vi "Find (Create) Object.vi"(7 "Object Path":string, 8 "error in (no error)":errorcluster, 10 "Starting Offset":i32, 11 "JSON":string) -> (0 "error out":errorcluster, 2 "Object offset":i32, 3 "<JSON>":string caption="<JSON> (possibly with empty object inserted)")   [LabVIEW 2015, in "JSONtext.lvlib"]
doc: "Ensures that a JSON Object exists at Path, and returns the offset to that object. If the object does not exist but it's parent object does, then an empty object is inserted. An error is output if a non-object exists at the specified path."
uses:
  JSONtext.lvlib
  Replace at Offset.vi
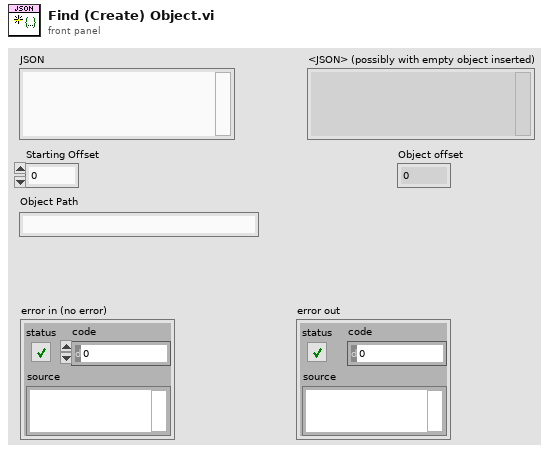
[diagram p1: front panel]
types:
  T1 = typedef "JSONtext.lvlib/Found Items.ctl" = cluster{"Item offset":i32, "Offset past Item":i32, "Name offset":i32, "Offset past Name":i32, "Found":bool, "Empty Object":bool}
  T2 = typedef "JSONtext.lvlib/Parsing State.ctl" = enum16{"Parser Error", "Object", "Array", "String", "Number/Other", "Leading Whitespace", "Object end", "Array end", "Value end"}
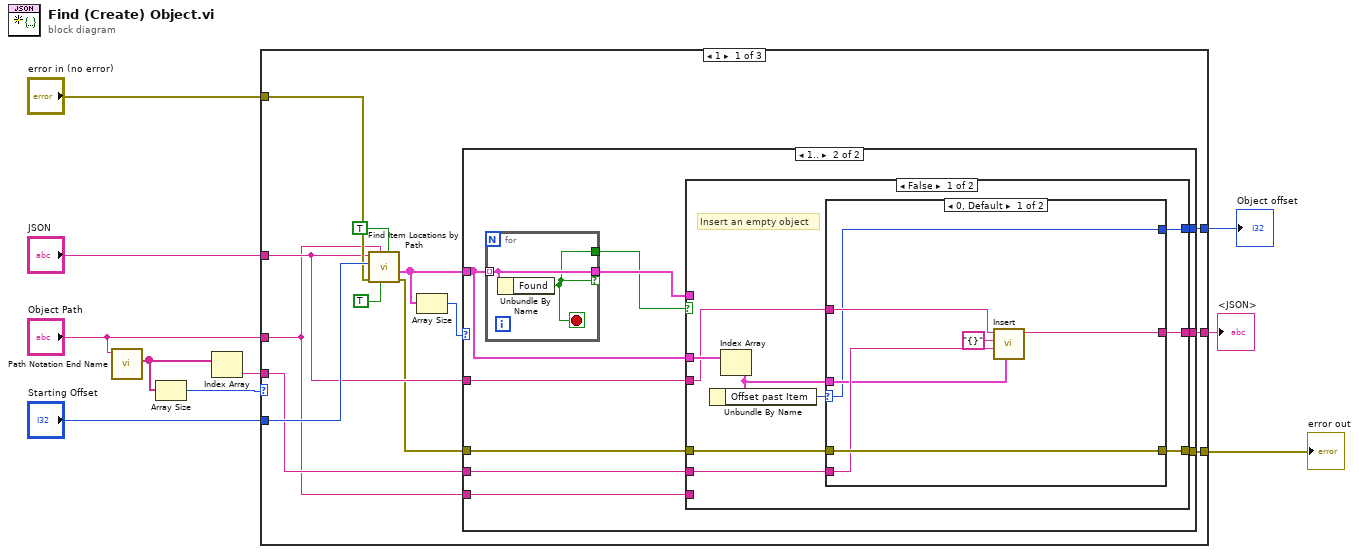
[diagram p0: block diagram]
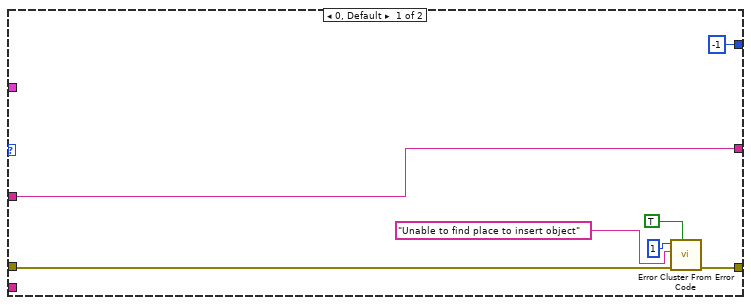
[diagram p2: hidden frame]
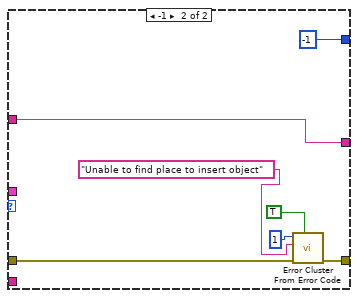
[diagram p3: hidden frame]
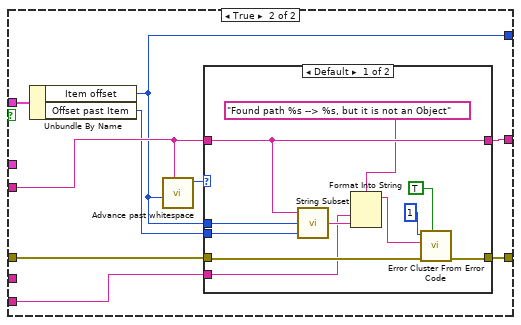
[diagram p4: hidden frame]
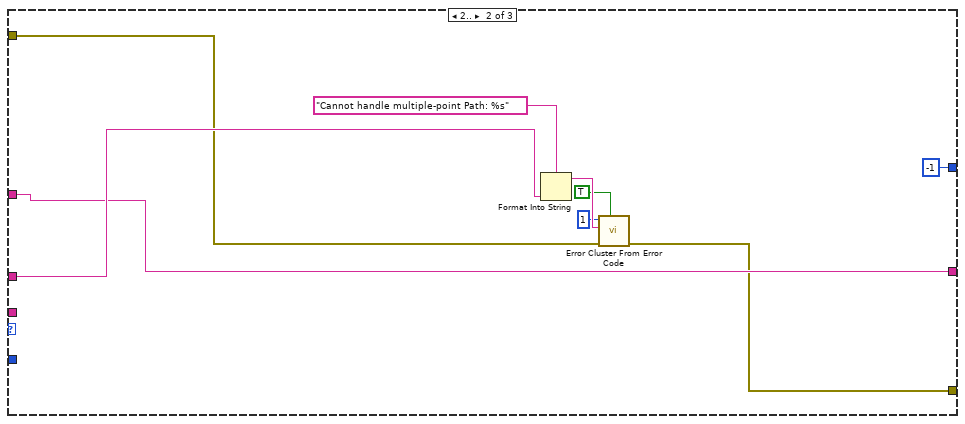
[diagram p6: hidden frame]
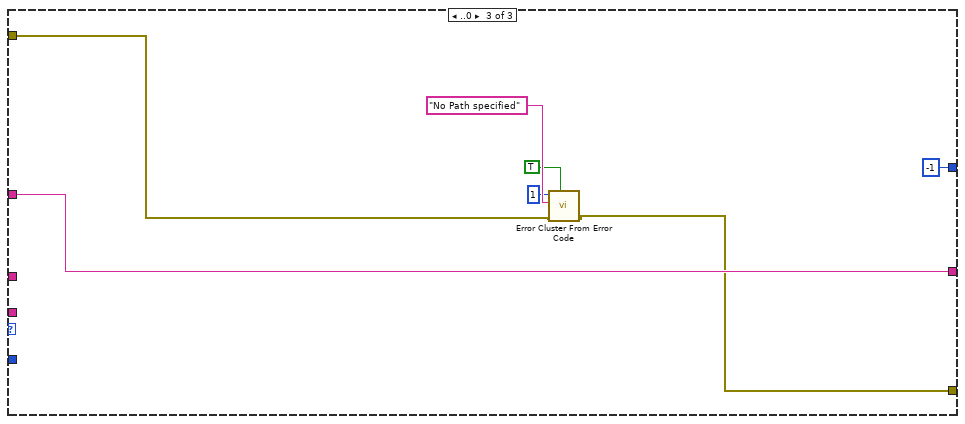
[diagram p7: hidden frame]
diagram:
  n1 = call "Path Notation End Name.vi"("Item Path"="Object Path") -> ("<JSON>End Names"=w5:string[])  [unwired: 10 in]
  n2 = Array Size(array=w5) -> (size(s)=w3:i32)
  n3 = Index Array(array=w5) -> (element=w2:string)  [unwired: 1 in]
  n4 = case shown="1" w3 {
    tunnel: "Object Path" -> [w13 w95 _]
    tunnel: "Starting Offset" -> [w23 _ _]
    tunnel: "error in (no error)" -> [w22 w89 w101]
    tunnel: [w16 w88 w100] -> w8
    tunnel: "JSON" -> [w21 w93 w102]
    tunnel: [w19 -1 ("Item offset") -1 ("Item offset")] -> w6
    tunnel: w2 -> [w15 _ _]
    tunnel: [w14 w93 w102] -> w1
    frame 1 {
      n5 = call "Find Item Locations by Path.vi"("Insertion point if not found"=TRUE, "Only return first found"=TRUE, "Path"=w13, "error in (no error)"=w22, "Object Offset"=w23, "JSON"=w21) -> ("error out"=w17:errorcluster, "Items"=w12:T1[])  [unwired: 4 in]
      n6 = Array Size(array=w12) -> (size(s)=w11:i32)
      n7 = case shown="1.." w11 {
        tunnel: w21 -> [w29 w40]
        tunnel: [-1 ("Item offset") w38] -> w19
        tunnel: w17 -> [w24 w36]
        tunnel: [w25 w35] -> w16
        tunnel: w15 -> [_ w34]
        tunnel: [w29 w33] -> w14
        tunnel: w13 -> [_ w32]
        tunnel: w12 -> [_ w31]
        frame 0, Default {
          n8 = call <vilib>:"Error Cluster From Error Code.vi"("show call chain? (False)"=TRUE, "error in (no error)"=w24, "error message (\"\")"="Unable to find place to insert object", "error code (0)"=1) -> ("error out"=w25:errorcluster)  [unwired: 5 in]
        }
        frame 1.. {
          n9 = for {
            tunnel: w31 -> [w42] mode=indexing
            tunnel: [w42] -> w39 if=w41
            tunnel: [w41] -> w37
            stop <- w41 stop-if-true
            n10 = Unbundle By Name(w42) -> ("Found"=w41:bool)
          }
          n11 = case shown="False" w37 {
            tunnel: w40 -> [w47 w69]
            tunnel: w39 -> [_ w74]
            tunnel: [w43 w68] -> w38
            tunnel: w36 -> [w48 w71]
            tunnel: [w49 w72] -> w35
            tunnel: w31 -> [w51 _]
            tunnel: w34 -> [w46 _]
            tunnel: [w44 w70] -> w33
            tunnel: w32 -> [_ w66]
            frame False {
              # "Insert an empty object"
              n12 = Index Array(array=w51) -> (element=w45:T1)  [unwired: 1 in]
              n13 = Unbundle By Name(w45) -> ("Offset past Item"=w50:i32)
              n14 = case shown="0, Default" w50 {
                selector: w50 -> [w52 _]
                tunnel: [w58 w65] -> w49
                tunnel: w48 -> [w58 w64]
                tunnel: w47 -> [w57 w60]
                tunnel: w46 -> [w56 _]
                tunnel: w45 -> [w54 _]
                tunnel: [w53 w60] -> w44
                tunnel: [w52 -1 ("Item offset")] -> w43
                frame 0, Default {
                  n15 = call "Insert.vi"("Item"=w54, "<JSON>name"=w56, "JSON to Insert"="{}", "JSON in"=w57) -> ("string"=w53:string)  [unwired: 6 in, 1 out]
                }
                frame -1 {
                  n16 = call <vilib>:"Error Cluster From Error Code.vi"("show call chain? (False)"=TRUE, "error in (no error)"=w64, "error message (\"\")"="Unable to find place to insert object", "error code (0)"=1) -> ("error out"=w65:errorcluster)  [unwired: 5 in]
                }
              }
            }
            frame True {
              n17 = Unbundle By Name(w74) -> ("Item offset"=w68:i32, "Offset past Item"=w67:i32)
              n18 = call "Advance past whitespace.vi"("JSON"=w69, "Offset"=w68) -> ("Parser State"=w73:T2)  [unwired: 8 in, 1 out]
              n19 = case shown="Default" w73 {
                tunnel: [w85 w87] -> w72
                tunnel: w71 -> [w84 w87]
                tunnel: [w81 w86] -> w70
                tunnel: w69 -> [w81 w86]
                tunnel: w68 -> [w80 _]
                tunnel: w67 -> [w79 _]
                tunnel: w66 -> [w75 _]
                frame Default {
                  n20 = call "String Subset.vi"("Offset past End"=w79, "Start offset"=w80, "JSON"=w81) -> ("substring"=w77:string)  [unwired: 2 in]
                  n21 = Format Into String(format string="Found path %s --> %s, but it is not an Object" ("error message (\"\")"), w75, w77) -> (resulting string=w76:string)  [unwired: 2 in, 1 out]
                  n22 = call <vilib>:"Error Cluster From Error Code.vi"("show call chain? (False)"=TRUE, "error in (no error)"=w84, "error message (\"\")"=w76, "error code (0)"=1) -> ("error out"=w85:errorcluster)  [unwired: 5 in]
                }
                frame "Object" {
                }
              }
            }
          }
        }
      }
    }
    frame 2.. {
      n23 = Format Into String(format string="Cannot handle multiple-point Path: %s", w95) -> (resulting string=w92:string)  [unwired: 2 in, 1 out]
      n24 = call <vilib>:"Error Cluster From Error Code.vi"("show call chain? (False)"=TRUE, "error in (no error)"=w89, "error message (\"\")"=w92, "error code (0)"=1) -> ("error out"=w88:errorcluster)  [unwired: 5 in]
    }
    frame ..0 {
      n25 = call <vilib>:"Error Cluster From Error Code.vi"("show call chain? (False)"=TRUE, "error in (no error)"=w101, "error message (\"\")"="No Path specified" ("format string"), "error code (0)"=1) -> ("error out"=w100:errorcluster)  [unwired: 5 in]
    }
  }
  "error out" <- w8
  "Object offset" <- w6
  "<JSON>" <- w1
